vi "getInstanceClassAttributes.vi"(5 "Address":string="localhost", 7 "Data Source":string, 8 "error in (no error)":errorcluster, 9 "timeout ms (5000)":i32=5000, 11 "Instance Name":string) -> (0 "error out":errorcluster, 1 "timed out":bool, 2 "Class Name":string, 3 "Class Attributes":string[][](array[string]))   [LabVIEW 2014, in "CS SQL Server.lvlib"]
doc: "This VI can be used to query the CS Configuration Database for attributes of an instance that belong to its class, but not parents or childs. It could be called e.g. from the constructor to initialize its corresponding attribute values."
uses:
  CS SQL Server.lvlib
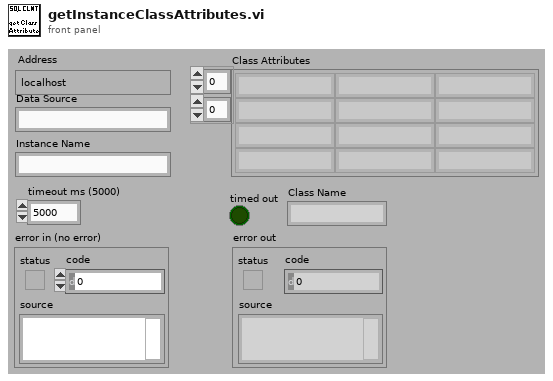
[diagram p1: front panel]
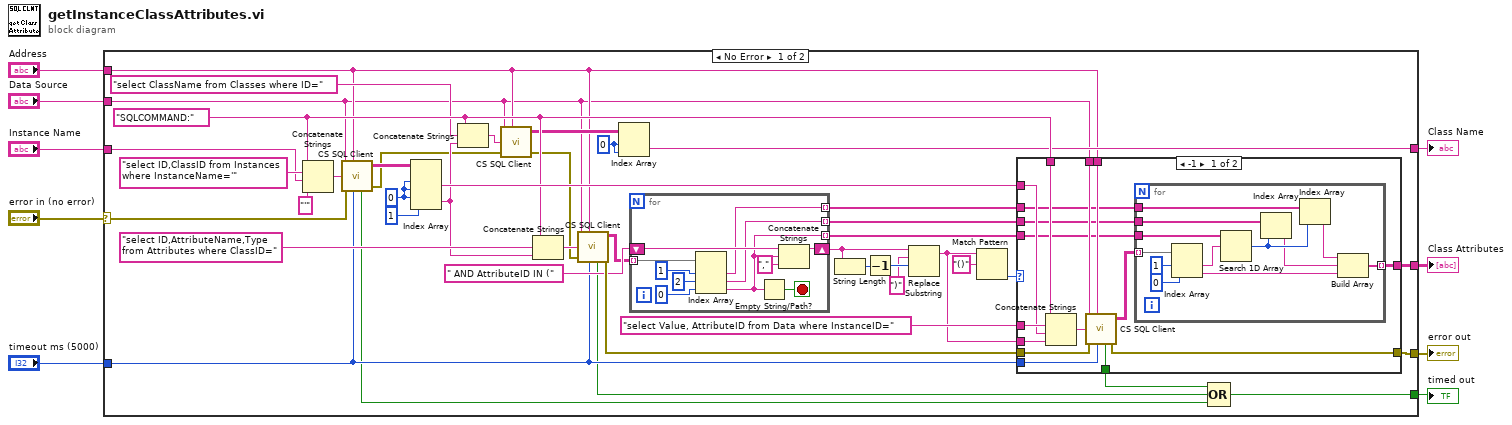
[diagram p0: block diagram]
diagram:
  n1 = case shown="No Error" "error in (no error)" {
    selector: "error in (no error)" -> [w24 w93]
    tunnel: "Data Source" -> [w10 _]
    tunnel: "Address" -> [w11 _]
    tunnel: "Instance Name" -> [w43 _]
    tunnel: [w35 _] -> w6
    tunnel: [w34 w93] -> w5
    tunnel: "timeout ms (5000)" -> [w29 _]
    tunnel: [w25 _] -> w3
    tunnel: [w12 _] -> w1
    frame No Error {
      w13 = 0 ("index (row)")
      w30 = 0 ("index (row)")
      w19 = "SQLCOMMAND:"
      n2 = Concatenate Strings(w19, "select ID,ClassID from Instances where InstanceName='" ("string"), w43, "'" ("string")) -> (w44:string)
      n3 = call "CS SQL Client.vi"("Data Source"=w10, "Address"=w11, "Process"=w44, "error in (no error)"=w24, "timeout ms (5000)"=w29) -> ("query results"=w32:string[][], "Timeout"=w27:bool, "error out"=w16:errorcluster)  [unwired: 2 out]
      n4 = Index Array(array=w32, index (row) #1=w30, index (col) #1=w30, index (row) #2=w30, index (col) #2=1 ("disabled index (col)")) -> (element #1=w31:string, element #2=w17:string)
      n5 = Concatenate Strings(w19, "select ClassName from Classes where ID=" ("string"), w17) -> (w20:string)
      n6 = call "CS SQL Client.vi"("Data Source"=w10, "Address"=w11, "Process"=w20, "error in (no error)"=w16) -> ("query results"=w14:string[][], "error out"=w15:errorcluster)  [unwired: 1 in, 3 out]
      n7 = Concatenate Strings(w19, "select ID,AttributeName,Type from Attributes where ClassID=" ("string"), w17) -> (w42:string)
      n8 = call "CS SQL Client.vi"("Data Source"=w10, "Address"=w11, "Process"=w42, "error in (no error)"=w15, "timeout ms (5000)"=w29) -> ("query results"=w45:string[][], "Timeout"=w26:bool, "error out"=w49:errorcluster)  [unwired: 2 out]
      n9 = Index Array(array=w14, index (row)=w13, index (col)=w13) -> (element=w12:string)
      n10 = for {
        tunnel: w45 -> [w92] mode=indexing
        shift-right: [w89] -> w38
        shift-left: " AND AttributeID IN (" -> [w91]
        tunnel: [w84] -> w23 mode=indexing
        tunnel: [w82] -> w22 mode=indexing
        tunnel: [w83] -> w21 mode=indexing
        stop <- w88 stop-if-true
        n11 = Index Array(array=w92, index #1=1 ("index"), index #2=2 ("index"), index #3=0 ("index")) -> (element #1=w83:string, element #2=w82:string, element #3=w84:string)
        n12 = Empty String/Path?(string/path=w84) -> (empty?=w88:bool)
        n13 = Concatenate Strings(w91, w84, "," ("string")) -> (w89:string)
      }
      n14 = String Length(string=w38) -> (length=w40:i32)
      n15 = Decrement(x=w40) -> (x-1=w41:i32)
      n16 = Replace Substring(3:w41, 4:")" ("substring (\"\")"), 5:w38) -> (1:w46:string)  [unwired: 2 out]
      n17 = Match Pattern(string=w46, regular expression="()") -> (offset past match=w37:i32)  [unwired: 4 out]
      n18 = case shown="-1" w37 {
        tunnel: "select Value, AttributeID from Data where InstanceID=" ("string") -> [w68 _]
        tunnel: w19 -> [w67 _]
        tunnel: w10 -> [w66 _]
        tunnel: w11 -> [w65 _]
        tunnel: w49 -> [w64 w81]
        tunnel: [w63 w81] -> w34
        tunnel: w31 -> [w60 _]
        tunnel: w46 -> [w61 _]
        tunnel: [w53 _] -> w35
        tunnel: w29 -> [w59 _]
        tunnel: [w58 _] -> w28
        tunnel: w23 -> [w56 _]
        tunnel: w22 -> [w55 _]
        tunnel: w21 -> [w54 _]
        frame -1 {
          n19 = Concatenate Strings(w67, w68, w60, w61) -> (w62:string)
          n20 = call "CS SQL Client.vi"("Data Source"=w66, "Address"=w65, "Process"=w62, "error in (no error)"=w64, "timeout ms (5000)"=w59) -> ("query results"=w57:string[][], "Timeout"=w58:bool, "error out"=w63:errorcluster)  [unwired: 2 out]
          n21 = for {
            tunnel: w57 -> [w80] mode=indexing
            tunnel: w56 -> [w78]
            tunnel: w55 -> [w76]
            tunnel: w54 -> [w75]
            tunnel: [w71] -> w53 mode=indexing
            n22 = Index Array(array=w80, index #1=1 ("index"), index #2=0 ("index")) -> (element #1=w77:string, element #2=w72:string)
            n23 = Search 1D Array(1D array=w78, element=w77) -> (index of element=w74:i32)  [unwired: 1 in]
            n24 = Index Array(array=w76, index=w74) -> (element=w69:string)
            n25 = Index Array(array=w75, index=w74) -> (element=w70:string)
            n26 = Build Array(w70, w69, w72) -> (w71:string[])
          }
        }
        frame Default {
          # "No AttributeID selected."
        }
      }
      n27 = Compound Arithmetic op=OR(w28, w26, w27) -> (w25:bool)
    }
    frame Error {
    }
  }
  "Class Attributes" <- w6
  "error out" <- w5
  "timed out" <- w3
  "Class Name" <- w1
